vi "Append Changed Items.vi"(6 "change type":T1, 7 "item name":string, 9 "items new":string[](array[string]), 10 "items old":string[](array[string]), 11 "refresh items in":T2[](array[typedef])) -> (2 "modify parent":bool, 3 "refresh items out":T2[](array[typedef]))   [LabVIEW 2020, in "AIM MIL-STD-1553 System Explorer.lvlib" / "Implementation.lvlib" / "Refresh.lvlib"]
uses:
  Refresh.lvlib
  MCL Row.ctl
  Change Type.ctl
  Symbols.ctl
  Name to Symbol.vi
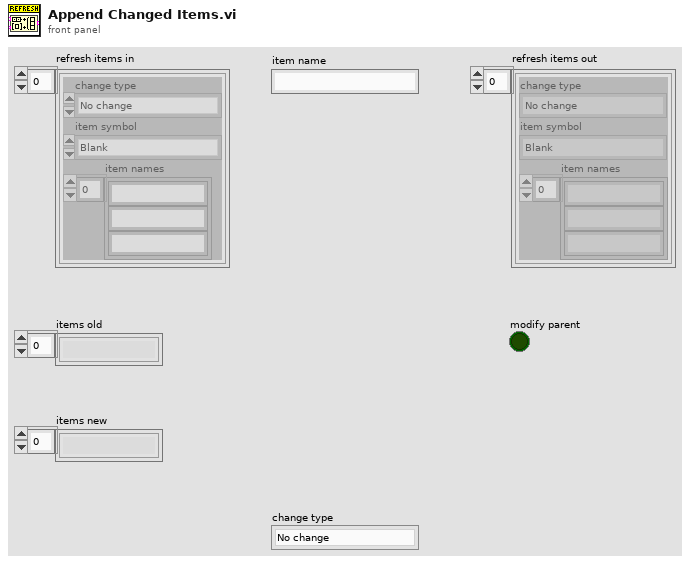
[diagram p1: front panel]
types:
  T1 = typedef "AIM MIL-STD-1553 System Explorer.lvlib/Implementation.lvlib/Refresh.lvlib/Change Type.ctl" = enum16{"No change", "Modify", "Add", "Remove"}
  T2 = typedef "AIM MIL-STD-1553 System Explorer.lvlib/Implementation.lvlib/Refresh.lvlib/MCL Row.ctl" = cluster{"change type":T1, "item symbol":T3, "item names":string[]}
  T3 = typedef "AIM MIL-STD-1553 System Explorer.lvlib/Implementation.lvlib/Refresh.lvlib/Symbols.ctl" = enum16{"Blank", "MIL-STD-1553", "Port", "Remote Terminal", "Subaddress", "Bus Controller", "Frame", "Mode Code", "Message", "Parameter", "Item"}
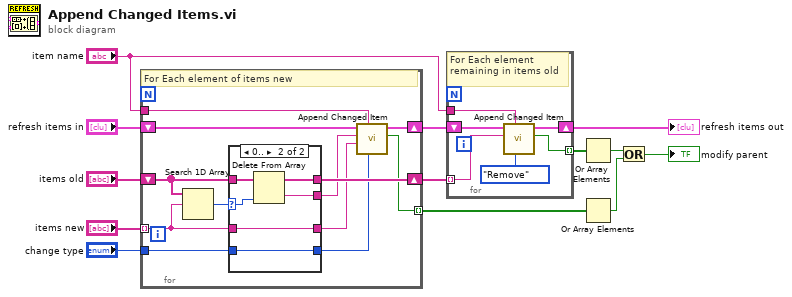
[diagram p0: block diagram]
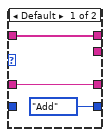
[diagram p2: hidden frame]
diagram:
  n1 = for {
    shift-right: [w23] -> w8
    shift-left: "items old" -> [w24]
    tunnel: "items new" -> [w22] mode=indexing
    shift-right: [w18] -> w12
    shift-left: "refresh items in" -> [w21]
    tunnel: "item name" -> [w17]
    tunnel: "change type" -> [w16]
    tunnel: [w14] -> w5 mode=indexing
    # "For Each element of items new"
    n2 = Search 1D Array(1D array=w24, element=w22) -> (index of element=w25:i32)  [unwired: 1 in]
    n3 = case shown="0.." w25 {
      selector: w25 -> [_ w34]
      tunnel: w24 -> [w28 w33]
      tunnel: [w28 w32] -> w23
      tunnel: w22 -> [w26 w31]
      tunnel: [w26 w31] -> w20
      tunnel: [Change_Type."Add" ("change type") w29] -> w15
      tunnel: [_ w30] -> w19
      tunnel: w16 -> [_ w29]
      frame Default {
      }
      frame 0.. {
        n4 = Delete From Array(array=w33, index=w34) -> (deleted portion=w30:string, array with subset deleted=w32:string[])  [unwired: 1 in]
      }
    }
    n5 = call "Append Changed Item.vi"("change type"=w15, "item name"=w17, "new value"=w20, "old value"=w19, "refresh items in"=w21) -> ("modify parent"=w14:bool, "refresh items out"=w18:T2[])  [unwired: 5 in]
  }
  n6 = for {
    tunnel: w8 -> [w37] mode=indexing
    shift-right: [w39] -> w7
    shift-left: w12 -> [w40]
    tunnel: "item name" -> [w36]
    tunnel: [w35] -> w4 mode=indexing
    # "For Each element remaining in items old"
    n7 = call "Append Changed Item.vi"("change type"=Change_Type."Remove", "item name"=w36, "old value"=w37, "refresh items in"=w40) -> ("modify parent"=w35:bool, "refresh items out"=w39:T2[])  [unwired: 6 in]
  }
  "refresh items out" <- w7
  n8 = Or Array Elements(Boolean array=w4) -> (logical OR=w3:bool)
  n9 = Or Array Elements(Boolean array=w5) -> (logical OR=w2:bool)
  n10 = Or(x=w3, y=w2) -> (x .or. y?=→"modify parent":bool)
